vi "Read Scaling Information.vi"(8 "error in":errorcluster, 11 "Input Channels in":refnum<class "Input Channels.lvclass">) -> (0 "error out":errorcluster, 2 "Scaling Information":T1, 3 "Input Channels out":refnum<class "Input Channels.lvclass">)   [LabVIEW 2020, in "Plugin.lvlib" / "Input Channels.lvclass"]
doc: "Reads Scaling Information."
uses:
  Input Channels.lvclass
  builds/Libraries/LabSys Framework.lvlibp/Configuration Storage/Test Configuration/Scaling Information.ctl
  builds/Libraries/LabSys Framework.lvlibp/Configuration Storage/Test Configuration/Scaling Types.ctl
  Input Channels.lvclass/Input Channels.ctl
  builds/Libraries/LabSys Framework.lvlibp/Configuration Storage/Test Configuration/Test Configuration.lvclass
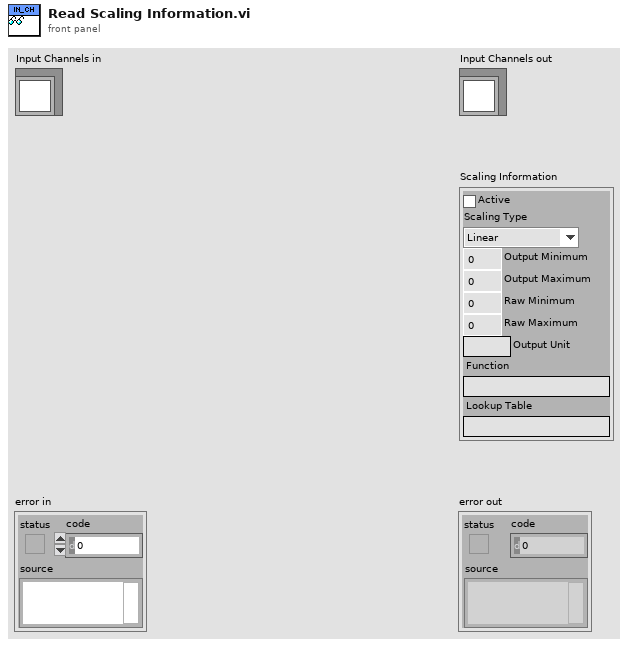
[diagram p1: front panel]
types:
  T1 = typedef "LabSys Framework.lvlibp/Configuration Storage.lvlib/Test Configuration.lvclass/Scaling Information.ctl" = cluster{"Active":bool, "Scaling Type":T2, "Output Minimum":dbl, "Output Maximum":dbl, "Raw Minimum":dbl, "Raw Maximum":dbl, "Output Unit":string, "Function":string, "Lookup Table":string}
  T2 = typedef "LabSys Framework.lvlibp/Configuration Storage.lvlib/Test Configuration.lvclass/Scaling Types.ctl" = enum8{"Linear", "Function", "Lookup Table"}
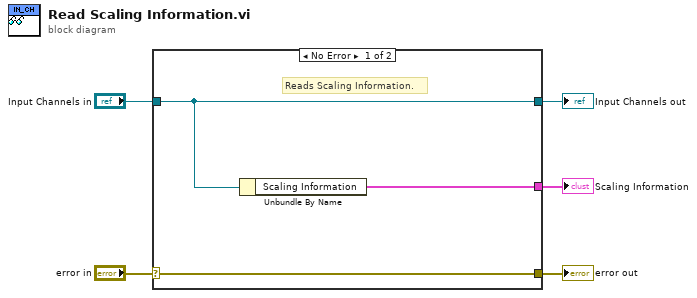
[diagram p0: block diagram]
diagram:
  n1 = case shown="No Error" "error in" {
    selector: "error in" -> [w8 w9]
    tunnel: [w8 w9] -> w4
    tunnel: [w7 w10] -> w2
    tunnel: "Input Channels in" -> [w7 w10]
    tunnel: [w6 _] -> w1
    frame No Error {
      # "Reads Scaling Information."
      n2 = Unbundle By Name(w7) -> ("Scaling Information"=w6:T1)
    }
    frame Error {
    }
  }
  "error out" <- w4
  "Input Channels out" <- w2
  "Scaling Information" <- w1
